vi "Actor Core.vi"(8 "error in":errorcluster, 11 "Caller in":refnum<class "Nested.lvclass">) -> (0 "error out":errorcluster, 3 "Actor out":refnum<class "Actor.lvclass">)   [LabVIEW 2020, in "Nested.lvlib" / "Nested.lvclass"]
doc: "(<B>Filename</B>: Actor Framework.lvlib:Actor.lvclass:Actor Core.vi)\n\nReceives messages to the actor, reacts to them, and initiates any error handling that may shut the actor down.\n\nDescendant classes may override this VI to append parallel tasks for the actor to complete while it handles messages. Overrides use the Call Parent Class Method node."
uses:
  Nested.lvclass
  <vilib>/ActorFramework/Actor/Actor.lvclass
  Nested.lvclass/Nested.ctl
  CallerInterface Messages/UpdateCallerDisplay Msg/UpdateCallerDisplay Msg.lvclass/UpdateCallerDisplay Msg.ctl
  <vilib>/ActorFramework/Message Enqueuer/Message Enqueuer.lvclass/Message Enqueuer.ctl
  <vilib>/ActorFramework/Message Enqueuer/Enqueue.vi
  CallerInterface Messages/UpdateCallerDisplay Msg/UpdateCallerDisplay Msg.lvclass
  C:/Program Files/National Instruments/LabVIEW 2020/vi.lib/ActorFramework/Message/Message.lvclass
  Nested Messages/Error Msg/Error Msg.lvclass
  <vilib>/ActorFramework/Stop Msg/Stop Msg.lvclass
  <vilib>/ActorFramework/Message Priority Queue/Priority Enqueue.vi
panel:
  in  "Btn_Error":bool
  in  "Message":string
  out "Display":string
  in  "Btn_ Sendmsg_Caller":bool
  # "Nested"
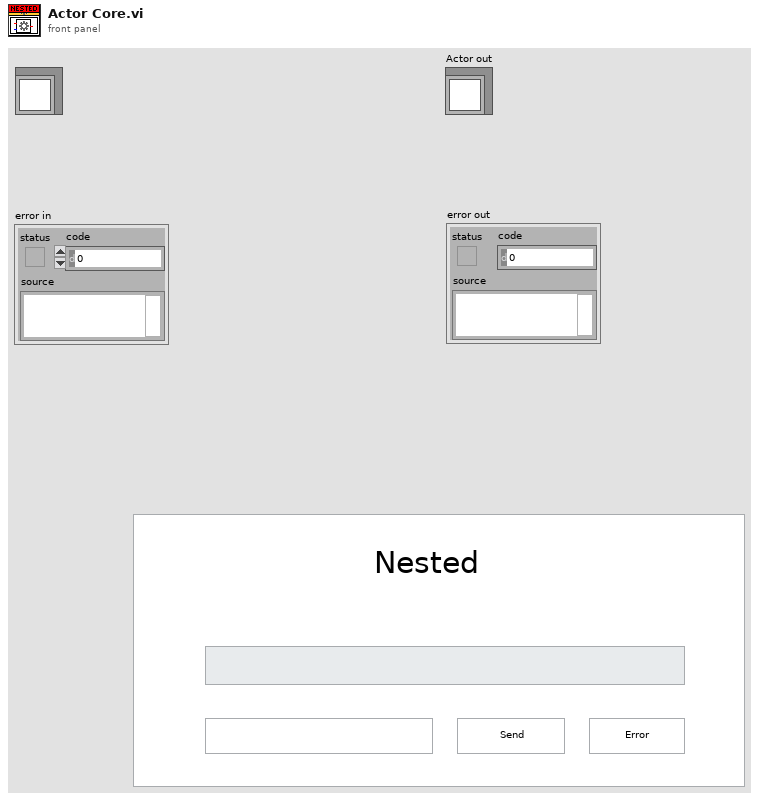
[diagram p1: front panel]
types:
  T1 = cluster{"Quit":refnum<user-event>, "Update Display":refnum<user-event>}
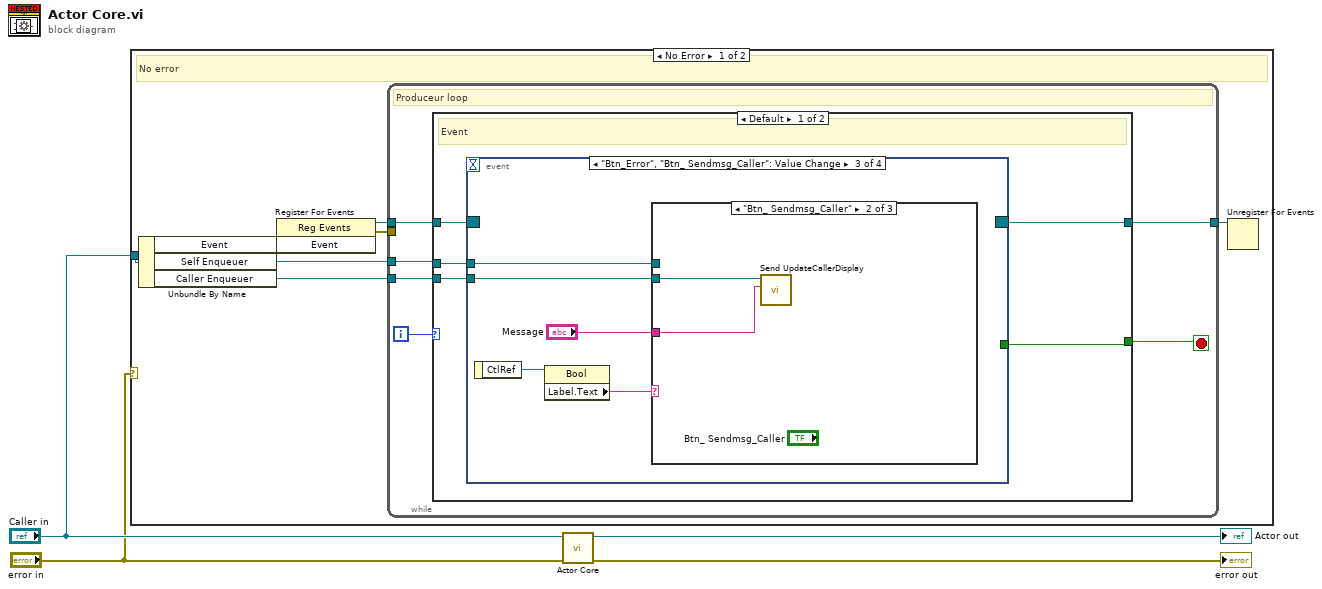
[diagram p0: block diagram]
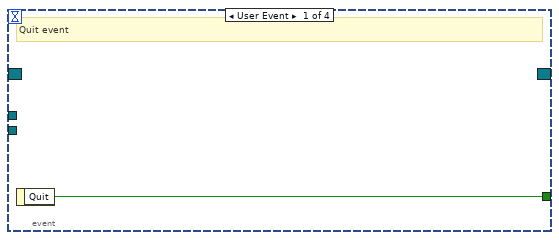
[diagram p2: hidden frame]
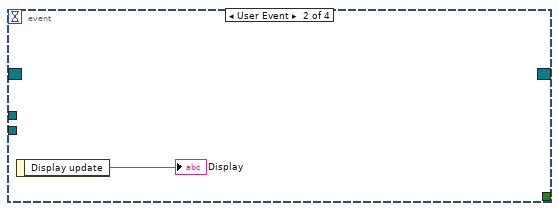
[diagram p3: hidden frame]
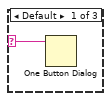
[diagram p4: hidden frame]
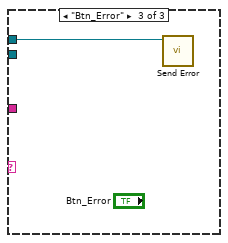
[diagram p5: hidden frame]
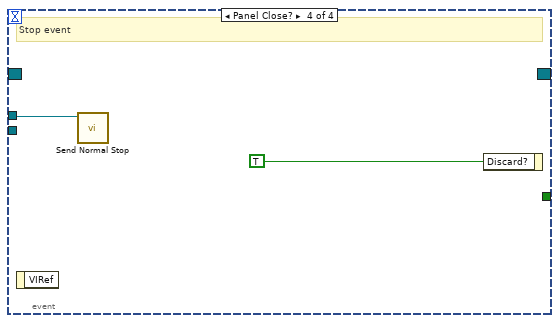
[diagram p6: hidden frame]
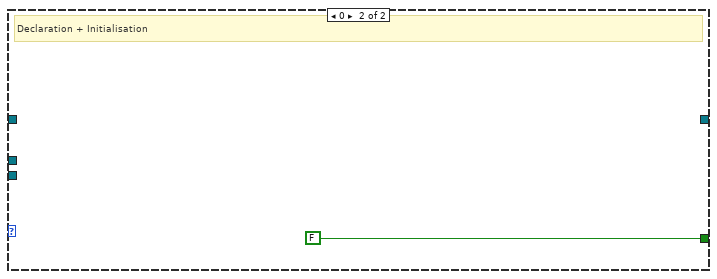
[diagram p7: hidden frame]
diagram:
  n1 = case shown="No Error" "error in" {
    tunnel: "Caller in" -> [w9 _]
    frame No Error {
      # "No error"
      n2 = Unbundle By Name(w9) -> ("Event"=w7:T1, "Self Enqueuer"=w10:refnum<class "Message Enqueuer.lvclass">, "Caller Enqueuer"=w5:refnum<class "Message Enqueuer.lvclass">)
      n3 = register-events(w7) -> (reference out=w8:refnum<event-registration>, error out=w6:errorcluster)  [unwired: 2 in]
      n4 = while {
        tunnel: [w15] -> w11
        tunnel: w10 -> [w14]
        tunnel: w8 -> [w13]
        tunnel: w6 -> [_]
        tunnel: w5 -> [w12]
        i -> [w17]
        stop <- w16 stop-if-true
        # "Produceur loop"
        n5 = case shown="Default" w17 {
          tunnel: w14 -> [w20 _]
          tunnel: [w21 FALSE] -> w16
          tunnel: [w22 _] -> w15
          tunnel: w13 -> [w19 _]
          tunnel: w12 -> [w18 _]
          frame Default {
            # "Event"
            n6 = event shown="[2] \"Btn_Error\", \"Btn_ Sendmsg_Caller\": Value Change" {
              selector: w19 -> [_ _ _ _]
              dyn-events: [_ _ _ _] -> w22
              timeout: _ -> [_ _ _ _]
              tunnel: [w23 _ _ _] -> w21
              tunnel: w20 -> [_ _ w27 w34]
              tunnel: w18 -> [_ _ w25 _]
              event User Event {
                # "Quit event"
                n7 = event-data() -> ("Quit"=w23:bool)  [unwired: 1 in]
              }
              event User Event {
                n8 = event-data() -> ("Display update"=→"Display":string)  [unwired: 1 in]
              }
              event "Btn_Error", "Btn_ Sendmsg_Caller": Value Change {
                n9 = event-data() -> ("CtlRef"=w29:refnum<vi>)  [unwired: 1 in]
                n10 = property class="Bool"(reference=w29) -> ("Label.Text"=w28:string)  [unwired: 1 in, 2 out]
                n11 = case shown="\"Btn_ Sendmsg_Caller\"" w28 {
                  selector: w28 -> [w30 _ _]
                  tunnel: w27 -> [_ _ w33]
                  tunnel: "Message" -> [_ w32 _]
                  tunnel: w25 -> [_ w31 _]
                  frame Default {
                    n12 = One Button Dialog(message=w30) -> ()  [unwired: 1 in, 1 out]
                  }
                  frame "Btn_ Sendmsg_Caller" {
                    n13 = call "Send UpdateCallerDisplay.vi"("Message"=w32, "Message Enqueuer"=w31) -> ()  [unwired: 8 in, 2 out]
                  }
                  frame "Btn_Error" {
                    n14 = call "Send Error.vi"("Message Enqueuer"=w33) -> ()  [unwired: 9 in, 2 out]
                  }
                }
              }
              event Panel Close? {
                # "Stop event"
                n15 = event-data() -> ()  [unwired: 1 in, 1 out]
                n16 = call <vilib>:"Send Normal Stop.vi"("Message Enqueuer"=w34) -> ()  [unwired: 10 in, 1 out]
                n17 = event-data("Discard?"=TRUE) -> ()  [unwired: 1 in, 1 out]
              }
            }
          }
          frame 0 {
            # "Declaration + Initialisation"
          }
        }
      }
      n18 = Unregister For Events(event registration refnum=w11) -> ()  [unwired: 1 in, 1 out]
    }
    frame Error {
    }
  }
  n19 = call-parent "Actor Core.vi"("error in"="error in", "Actor in"="Caller in") -> ("error out"=→"error out":errorcluster, "Actor out"=→"Actor out":refnum<class "Actor.lvclass">)  [unwired: 8 in]
